vi "NavX Query.vi"   [LabVIEW 2017]
uses:
  <vilib>/Rock Robotics/Network Tables/NT Read Boolean.vi
  <vilib>/Rock Robotics/Network Tables/NT Write Number.vi
types:
  T1 = cluster{"Yaw":dbl, "Roll":dbl, "Pitch":dbl, "Heading":dbl, "Fused Heading":dbl}
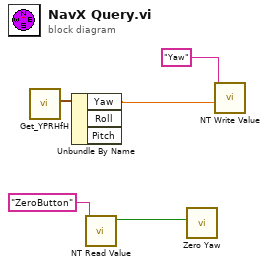
[diagram p0: block diagram]
diagram:
  n1 = call <vilib>:"Get_YPRHfH.vi"() -> ("YRPHfH"=w5:T1)  [unwired: 11 in]
  n2 = Unbundle By Name(w5) -> ("Yaw"=w3:dbl)  [unwired: 2 out]
  n3 = call-poly <vilib>:"NT Read Value.vi"("Name"="ZeroButton") -> ("Boolean"=w1:bool)  [unwired: 9 in, 1 out]
  n4 = call <vilib>:"Zero Yaw.vi"("Zero"=w1) -> ()  [unwired: 11 in]
  n5 = call-poly <vilib>:"NT Write Value.vi"("Numeric"=w3, "Name"="Yaw") -> ()  [unwired: 9 in, 1 out]
